vi "NumArray_to_SpdshtStr_prepend.vi"(9 "Column headers":string[](array[string])=["Time/s", "TH/Celsius", "TC/Celsius", "Delta V"]) -> (1 "concatenated string":string)   [LabVIEW 2015]
panel:
  in  "delimiter (Tab) 2":string
  out "spreadsheet string":string
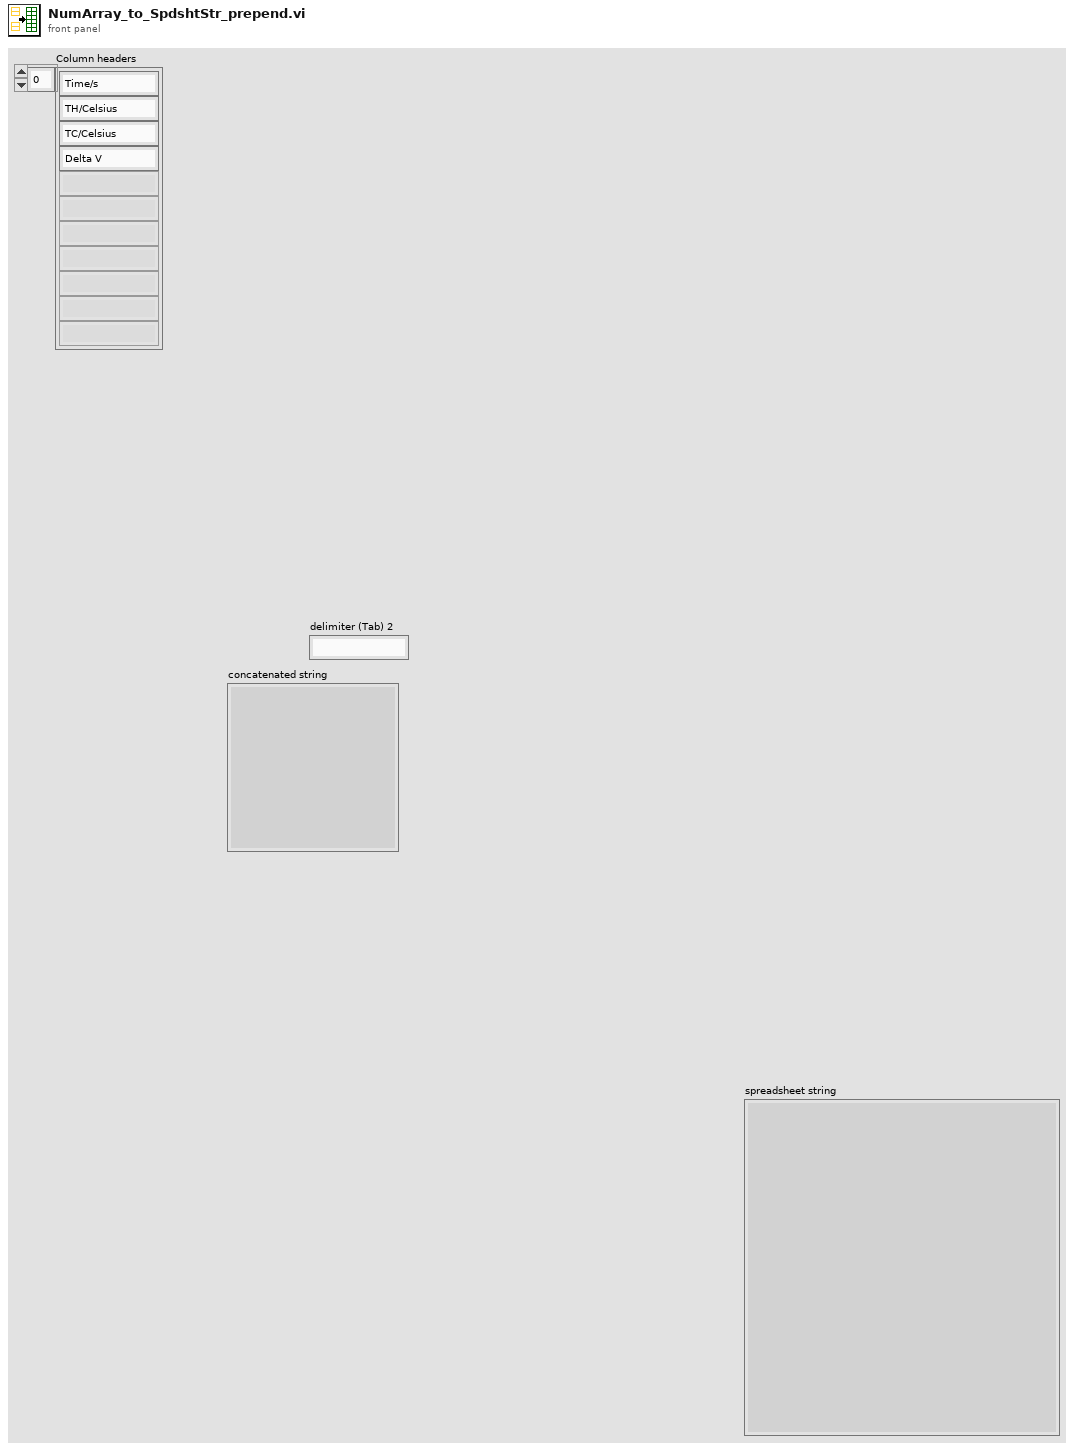
[diagram p1: front panel]
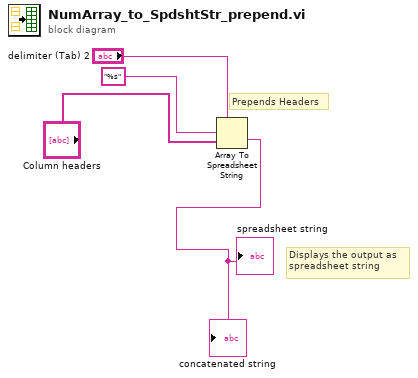
[diagram p0: block diagram]
diagram:
  # "Displays the output as \nspreadsheet string"
  # "Prepends Headers"
  n1 = Array To Spreadsheet String(delimiter (Tab)="delimiter (Tab) 2", array="Column headers", 3:"%s" ("format string")) -> (spreadsheet string=→"spreadsheet string" →"concatenated string":string)
